vi "Sequence.Test.Load.vi"(7 "Code in":T1={"Ready"=FALSE, "DoubleOrder"=FALSE, "OrderDone"=FALSE, "AllowSingleSlot"=FALSE, "CheckDM"=FALSE, "ThresholdA"=0, "ThresholdB"=0, "Plate"=enum."Wabco", "ImgPath"=path "", "Variant"={"State"=enum."Init", "ImgPath"=path "", "WabcoPlate"="", "WabcoProduct"="", "ClientProduct"="", "ClientPlate"="", "TotalQuantity"=0, "OrderQuantity"=0, "Serial"=0, "Wabco"={"LaserJob"="", "AdditionalTxt"="037", "FactoryCode"="", "RevID"=0, "ForkID"=0, "FailuresLimit"=0, "GlobalCnt"=0, "Bank"=0, "SerialFormat"=enum."6 dig", "CoordA"={"X"=0.0, "Y"=0.0, "Angle"=0.0}, "CoordB"={"X"=0.0, "Y"=0.0, "Angle"=0.0}, "DMCconfig"=0}, "Client"={"LaserJob"="", "AdditionalTxt"="", "FactoryCode"="037", "RevID"=0, "ForkID"=0, "FailuresLimit"=0, "GlobalCnt"=0, "Bank"=0, "SerialFormat"=enum."6 dig", "CoordA"={"X"=0.0, "Y"=0.0, "Angle"=0.0}, "CoordB"={"X"=0.0, "Y"=0.0, "Angle"=0.0}, "DMCconfig"=0}}}, 8 "error in":errorcluster, 9 "#products in the machine":i32, 11 "Data in":T8) -> (0 "error out":errorcluster, 3 "Data out":T8)   [LabVIEW 2016]
uses:
  Sequence.Test.Status.ctl
  Sequence.Slot.StatusData.ctl
  Sequence.Test.Unload.Status.ctl
  Sequence.Prod.StatusData.ctl
  Sequence.Step.Status.ctl
  Sequence.Test.BreakReason.ctl
  Sequence.Code.Sets.ctl
  Sequence.PlateType.ctl
  Logger/Logger.Variant.Sets.ctl
  Station/Station.Changeover.State.vi
  Station/Station.Plate.Properties.ctl
  Sequence.Code.SerialFormat.ctl
  Drivers/V7310/LowLevel/V7310.Job.Sets.ctl
  Station/Station.ValvePosition.ctl
  Station/Station.ProductSlot.ctl
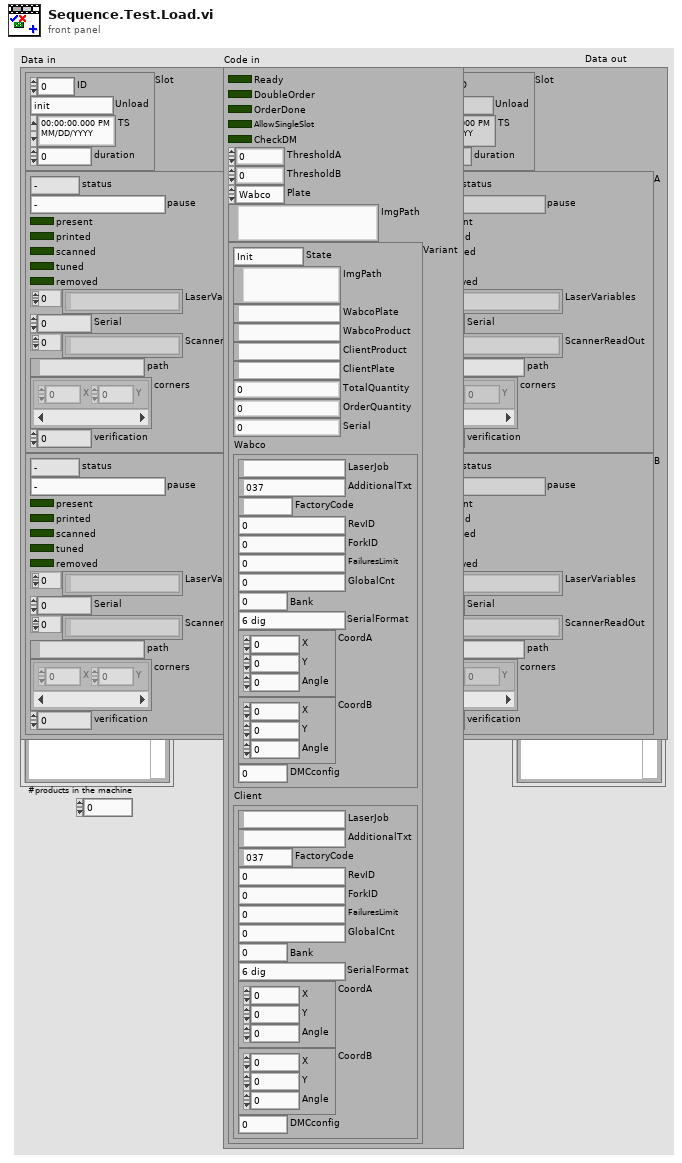
[diagram p1: front panel]
types:
  T1 = typedef "Sequence.Code.Sets.ctl" = cluster{"Ready":bool, "DoubleOrder":bool, "OrderDone":bool, "AllowSingleSlot":bool, "CheckDM":bool, "ThresholdA":u8, "ThresholdB":u8, "Plate":T2, "ImgPath":path, "Variant":T3}
  T2 = typedef "Sequence.PlateType.ctl" = enum16{"Wabco", "Client"}
  T3 = typedef "Logger.Variant.Sets.ctl" = cluster{"State":T4, "ImgPath":path, "WabcoPlate":string, "WabcoProduct":string, "ClientProduct":string, "ClientPlate":string, "TotalQuantity":u16, "OrderQuantity":u16, "Serial":i32, "Wabco":T5, "Client":T5}
  T4 = typedef "Station.Changeover.State.vi" = enum16{"Init", "Scaning", "NOK", "Wait for ack", "Ready"}
  T5 = typedef "Station.Plate.Properties.ctl" = cluster{"LaserJob":string, "AdditionalTxt":string, "FactoryCode":string, "RevID":u8, "ForkID":u8, "FailuresLimit":u16, "GlobalCnt":i32, "Bank":u8, "SerialFormat":T6, "CoordA":T7, "CoordB":T7, "DMCconfig":i32}
  T6 = typedef "Sequence.Code.SerialFormat.ctl" = enum8{"", "6 dig", "7 dig"}
  T7 = typedef "V7310.Job.Sets.ctl" = cluster{"X":dbl, "Y":dbl, "Angle":dbl}
  T8 = typedef "Sequence.Test.Status.ctl" = cluster{"Slot":T9, "A":T11, "B":T11}
  T9 = typedef "Sequence.Slot.StatusData.ctl" = cluster{"ID":i32, "Unload":T10, "TS":timestamp, "duration":u32}
  T10 = typedef "Sequence.Test.Unload.Status.ctl" = enum16{"init", "check NOK", "check OK", "wait on NOK", "wait on OK", "wait on Unload", "done"}
  T11 = typedef "Sequence.Prod.StatusData.ctl" = cluster{"status":T12, "pause":T13, "present":bool, "printed":bool, "scanned":bool, "tuned":bool, "removed":bool, "LaserVariables":string[], "Serial":i32, "ScannerReadOut":string[], "path":path, "corners":cluster{"X":i32, "Y":i32}[], "verification":u8}
  T12 = typedef "Sequence.Step.Status.ctl" = enum16{"-", "Pending", "Running", "Skipped", "Passed", "Failed", "Done", "Error", "Aborted", "Stopped"}
  T13 = typedef "Sequence.Test.BreakReason.ctl" = enum16{"-", "NOK container", "OK container", "Rev empty", "Rev missing", "Rev wrong", "Fork missing", "Fork wrong", "NOK limit", "Unload failure", "Single slot", "Part done", "Err: Prod move work", "Err: Prod move home", "Err: Prod lift work", "Err: Prod lift home", "Err: Prod Arm Work", "Err: Prod Arm NOK", "Err: Prod Arm OK", "Err: Prod NOK suck", "Err: Prod NOK drop", "Err: Prod OK missing", "Err: Prod OK suck", "Err: Prod OK drop"}
  T14 = typedef "Station.ValvePosition.ctl" = enum16{"Home", "Work"}
  T15 = typedef "FestoCPX.Station.RevolverID.ctl" = cluster{"ID":u8, "1":bool, "2":bool, "3":bool, "4":bool, "5":bool}
  T16 = typedef "Station.ProductSlot.ctl" = enum8{"A", "B"}
  T17 = typedef "Sequence.SerialsFglb.StatusFlags.ctl" = cluster{"Global":bool, "NokLimit":bool, "PartDone":bool, "Completed":bool}
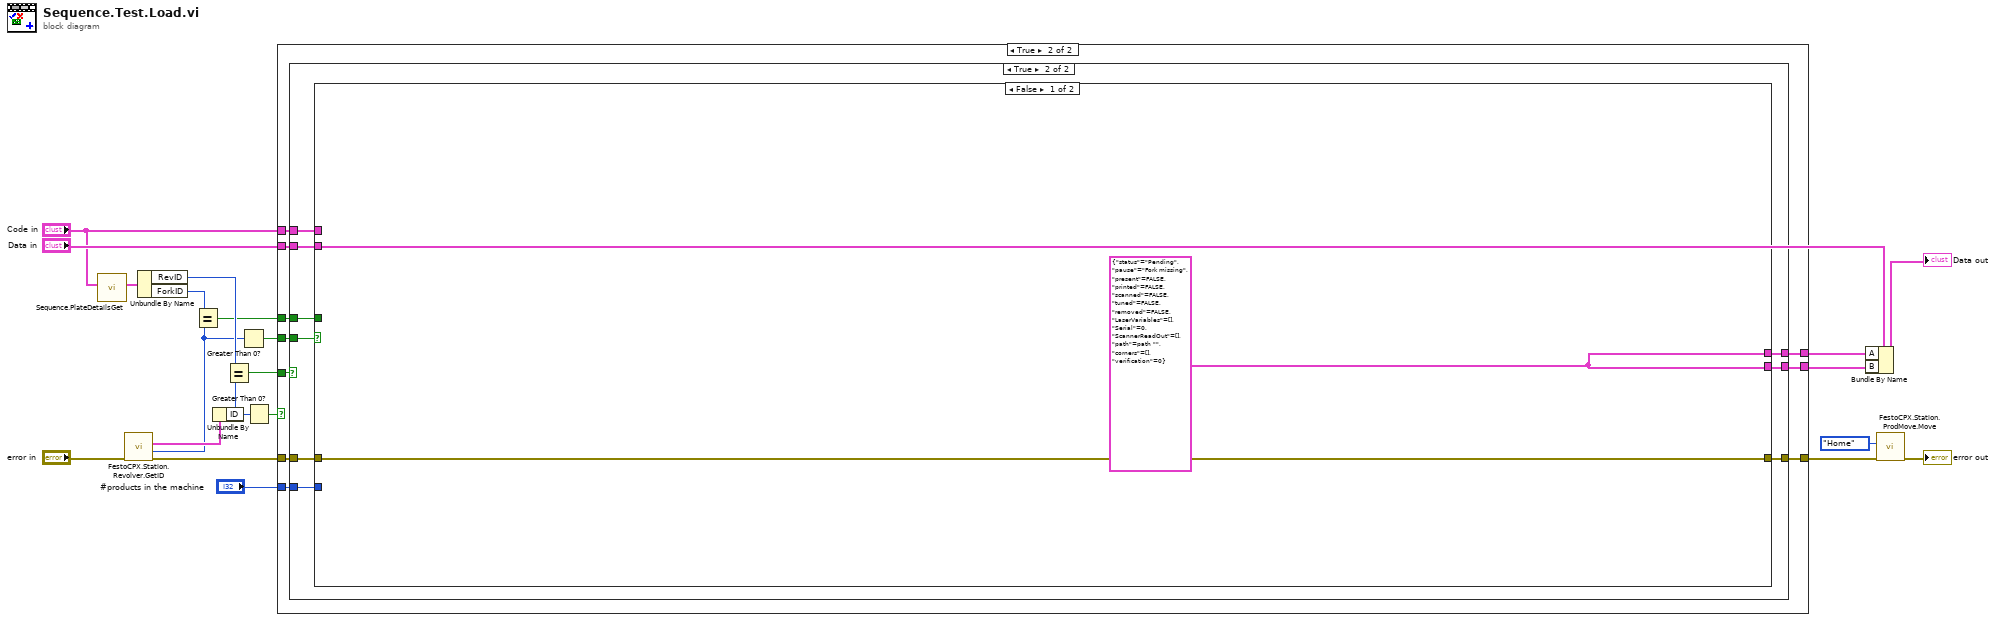
[diagram p0: block diagram]
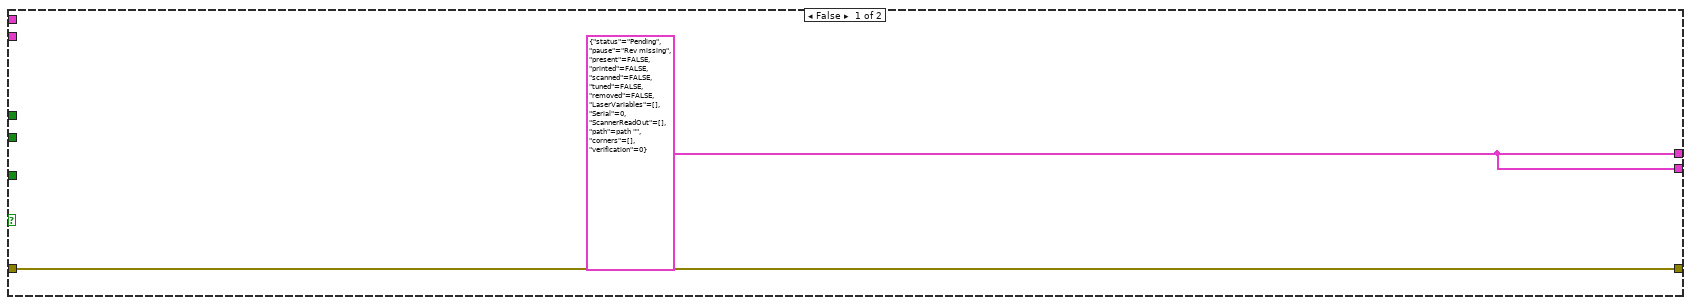
[diagram p2: hidden frame]
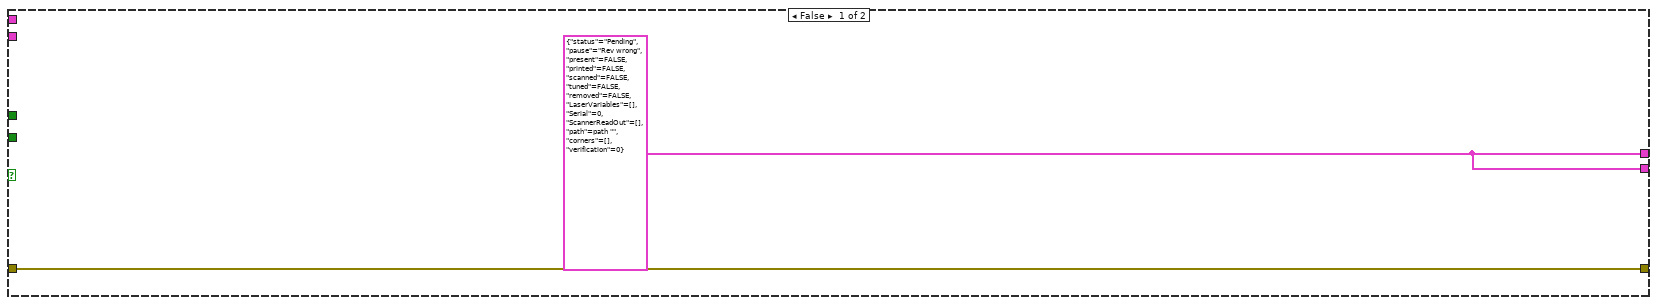
[diagram p3: hidden frame]
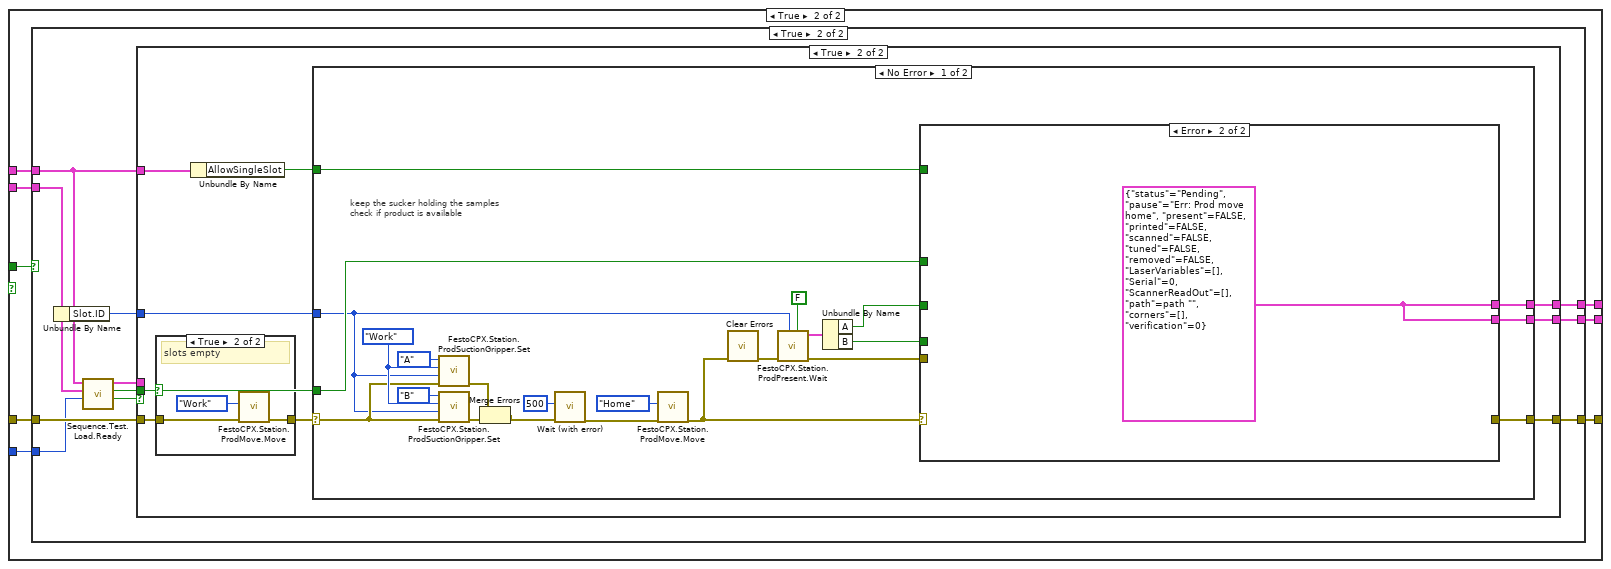
[diagram p4: hidden frame]
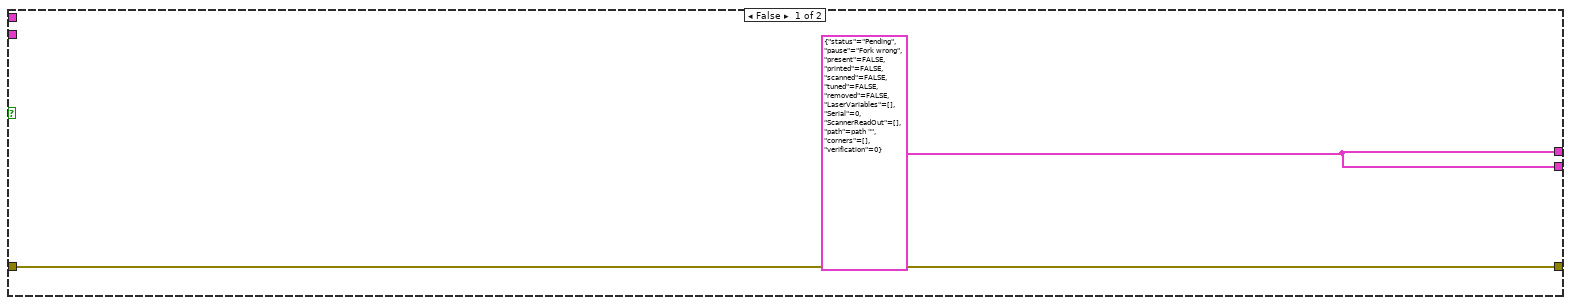
[diagram p5: hidden frame]
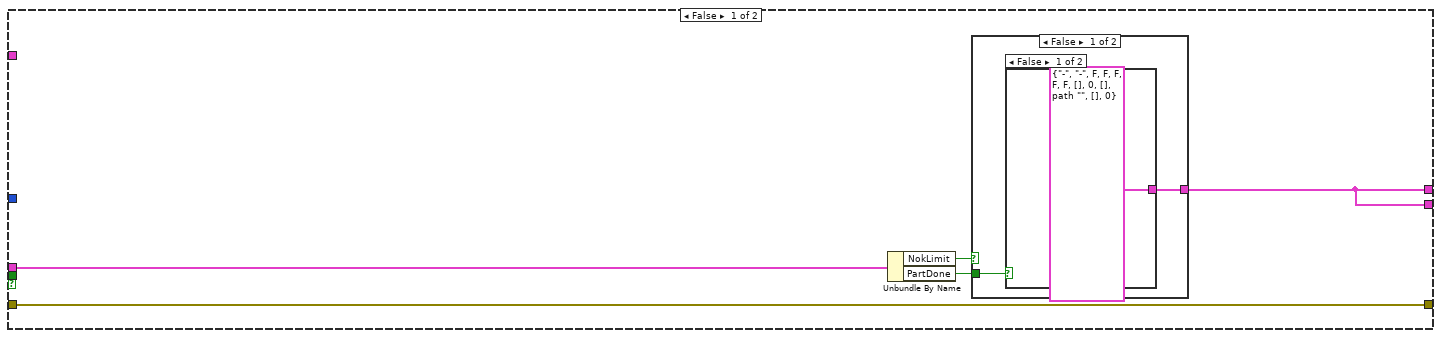
[diagram p6: hidden frame]
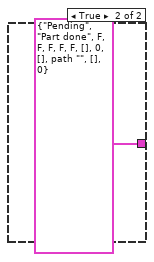
[diagram p7: hidden frame]
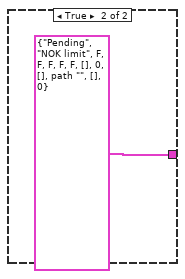
[diagram p8: hidden frame]
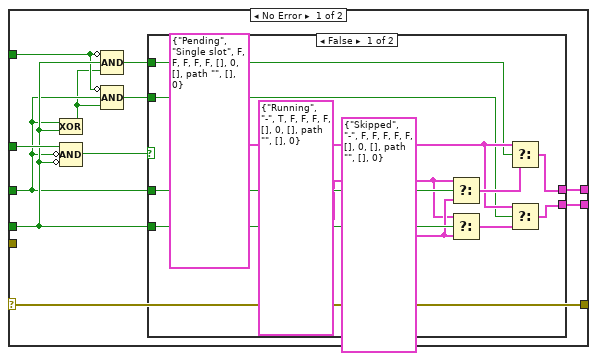
[diagram p9: hidden frame]
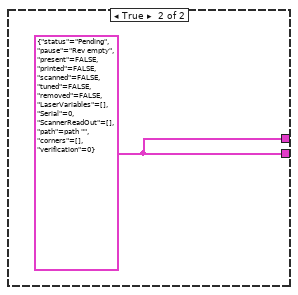
[diagram p10: hidden frame]
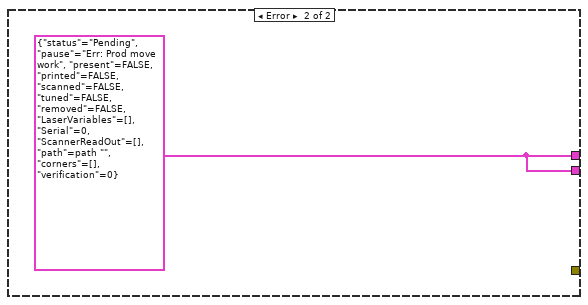
[diagram p11: hidden frame]
diagram:
  n1 = call "Sequence.PlateDetailsGet.vi"("Code in"="Code in") -> ("PlateDetails"=w3:T5)  [unwired: 9 in, 1 out]
  n2 = call "FestoCPX.Station.Revolver.GetID.vi"("error in"="error in") -> ("error out"=w16:errorcluster, "ForkID"=w8:u8, "RevID"=w15:T15)  [unwired: 8 in]
  n3 = Unbundle By Name(w3) -> ("RevID"=w10:u8, "ForkID"=w11:u8)
  n4 = Equal?(x=w11, y=w8) -> (x = y?=w9:bool)
  n5 = Unbundle By Name(w15) -> ("ID"=w13:u8)
  n6 = Equal?(x=w10, y=w13) -> (x = y?=w12:bool)
  n7 = Greater Than 0?(x=w8) -> (x > 0?=w7:bool)
  n8 = Greater Than 0?(x=w13) -> (x > 0?=w14:bool)
  n9 = case shown="True" w14 {
    tunnel: [w23 w33] -> w20
    tunnel: [w23 w32] -> w19
    tunnel: [w22 w31] -> w5
    tunnel: "Data in" -> [_ w30]
    tunnel: "Code in" -> [_ w29]
    tunnel: w16 -> [w22 w28]
    tunnel: w12 -> [_ w27]
    tunnel: w9 -> [_ w26]
    tunnel: w7 -> [_ w25]
    tunnel: "#products in the machine" -> [_ w24]
    frame False {
      w23 = T11 {"status"=enum."Pending", "pause"=enum."Rev missing", "present"=FALSE, "printed"=FALSE, "scanned"=FALSE, "tuned"=FALSE, "removed"=FALSE, "LaserVariables"=[], "Serial"=0, "ScannerReadOut"=[], "path"=path "", "corners"=[], "verification"=0} ("A")
    }
    frame True {
      n10 = case shown="True" w27 {
        tunnel: [w35 w44] -> w33
        tunnel: [w35 w43] -> w32
        tunnel: [w34 w42] -> w31
        tunnel: w30 -> [_ w41]
        tunnel: w29 -> [_ w39]
        tunnel: w28 -> [w34 w40]
        tunnel: w26 -> [_ w38]
        tunnel: w25 -> [_ w37]
        tunnel: w24 -> [_ w36]
        frame False {
          w35 = T11 {"status"=enum."Pending", "pause"=enum."Rev wrong", "present"=FALSE, "printed"=FALSE, "scanned"=FALSE, "tuned"=FALSE, "removed"=FALSE, "LaserVariables"=[], "Serial"=0, "ScannerReadOut"=[], "path"=path "", "corners"=[], "verification"=0} ("A")
        }
        frame True {
          n11 = case shown="False" w37 {
            tunnel: [w46 w54] -> w44
            tunnel: [w46 w53] -> w43
            tunnel: [w45 w52] -> w42
            tunnel: w41 -> [_ w51]
            tunnel: w40 -> [w45 w50]
            tunnel: w39 -> [_ w49]
            tunnel: w38 -> [_ w48]
            tunnel: w36 -> [_ w47]
            frame False {
              w46 = T11 {"status"=enum."Pending", "pause"=enum."Fork missing", "present"=FALSE, "printed"=FALSE, "scanned"=FALSE, "tuned"=FALSE, "removed"=FALSE, "LaserVariables"=[], "Serial"=0, "ScannerReadOut"=[], "path"=path "", "corners"=[], "verification"=0} ("A")
            }
            frame True {
              n12 = case shown="True" w48 {
                tunnel: [w56 w67] -> w54
                tunnel: [w56 w66] -> w53
                tunnel: [w55 w65] -> w52
                tunnel: w51 -> [_ w63]
                tunnel: w50 -> [w55 w62]
                tunnel: w49 -> [_ w59]
                tunnel: w47 -> [_ w57]
                frame False {
                  w56 = T11 {"status"=enum."Pending", "pause"=enum."Fork wrong", "present"=FALSE, "printed"=FALSE, "scanned"=FALSE, "tuned"=FALSE, "removed"=FALSE, "LaserVariables"=[], "Serial"=0, "ScannerReadOut"=[], "path"=path "", "corners"=[], "verification"=0} ("A")
                }
                frame True {
                  n13 = Unbundle By Name(w63) -> ("Slot.ID"=w64:i32)
                  n14 = call "Sequence.Test.Load.Ready.vi"("#products in the machine"=w57, "Data in"=w63, "Code in"=w59) -> ("Ready"=w61:bool, "Loaded"=w60:bool, "StatusFlags"=w58:T17)  [unwired: 6 in]
                  n15 = case shown="True" w61 {
                    tunnel: [w72 w86] -> w67
                    tunnel: [w72 w85] -> w66
                    tunnel: [w69 w78] -> w65
                    tunnel: w64 -> [_ w82]
                    tunnel: w62 -> [w69 w84]
                    tunnel: w60 -> [_ w83]
                    tunnel: w59 -> [_ w81]
                    tunnel: w58 -> [w68 _]
                    frame False {
                      n16 = Unbundle By Name(w68) -> ("NokLimit"=w71:bool, "PartDone"=w70:bool)
                      n17 = case shown="False" w71 {
                        tunnel: [w74 T11 {"status"=enum."Pending", "pause"=enum."NOK limit", "present"=FALSE, "printed"=FALSE, "scanned"=FALSE, "tuned"=FALSE, "removed"=FALSE, "LaserVariables"=[], "Serial"=0, "ScannerReadOut"=[], "path"=path "", "corners"=[], "verification"=0} ("A")] -> w72
                        tunnel: w70 -> [w73 _]
                        frame False {
                          n18 = case shown="False" w73 {
                            tunnel: [T11 {"status"=enum."-", "pause"=enum."-", "present"=FALSE, "printed"=FALSE, "scanned"=FALSE, "tuned"=FALSE, "removed"=FALSE, "LaserVariables"=[], "Serial"=0, "ScannerReadOut"=[], "path"=path "", "corners"=[], "verification"=0} ("A") T11 {"status"=enum."Pending", "pause"=enum."Part done", "present"=FALSE, "printed"=FALSE, "scanned"=FALSE, "tuned"=FALSE, "removed"=FALSE, "LaserVariables"=[], "Serial"=0, "ScannerReadOut"=[], "path"=path "", "corners"=[], "verification"=0} ("A")] -> w74
                            frame False {
                            }
                            frame True {
                            }
                          }
                        }
                        frame True {
                        }
                      }
                    }
                    frame True {
                      n19 = case shown="True" w83 {
                        tunnel: w84 -> [w135 w137]
                        tunnel: [w135 w136] -> w79
                        frame False {
                          # "product already loaded"
                        }
                        frame True {
                          # "slots empty"
                          n20 = call "FestoCPX.Station.ProdMove.Move.vi"("error in"=w137, "Position"=Station.ValvePosition."Work") -> ("error out"=w136:errorcluster)  [unwired: 8 in, 1 out]
                        }
                      }
                      n21 = Unbundle By Name(w81) -> ("AllowSingleSlot"=w80:bool)
                      n22 = case shown="No Error" w79 {
                        selector: w79 -> [w94 _]
                        tunnel: [w109 w134] -> w86
                        tunnel: [w108 w134] -> w85
                        tunnel: w83 -> [w104 _]
                        tunnel: w82 -> [w90 _]
                        tunnel: w80 -> [w93 _]
                        tunnel: [w95 _] -> w78
                        frame No Error {
                          w105 = Station.ValvePosition."Work" ("Position")
                          # "keep the sucker holding the samples\ncheck if product is available"
                          n23 = call "FestoCPX.Station.ProdSuctionGripper.Set.vi"("error in"=w94, "Sucker (0: Final)"=w90, "Position"=w105, "Slot"=Station.ProductSlot."A") -> ("error out"=w103:errorcluster)  [unwired: 6 in, 1 out]
                          n24 = call "FestoCPX.Station.ProdSuctionGripper.Set.vi"("error in"=w94, "Sucker (0: Final)"=w90, "Position"=w105, "Slot"=Station.ProductSlot."B") -> ("error out"=w102:errorcluster)  [unwired: 6 in, 1 out]
                          n25 = Merge Errors(w103, w102) -> (w89:errorcluster)
                          n26 = call "Wait (with error).vi"("error in (no error)"=w89, "milliseconds to wait"=u32 500) -> ("error out"=w97:errorcluster)  [unwired: 8 in, 1 out]
                          n27 = call "FestoCPX.Station.ProdMove.Move.vi"("error in"=w97, "Position"=Station.ValvePosition."Home") -> ("error out"=w87:errorcluster)  [unwired: 8 in, 1 out]
                          n28 = call <vilib>:"Clear Errors.vi"("error in (no error)"=w87) -> ("error out"=w96:errorcluster)  [unwired: 5 in, 1 out]
                          n29 = call "FestoCPX.Station.ProdPresent.Wait.vi"("AllowSingleSlot"=FALSE, "SuckerID (0: Final)"=w90, "error in"=w96) -> ("error out"=w91:errorcluster, "Present.SuckerID"=w100:cluster{"A":bool, "B":bool})  [unwired: 7 in]
                          n30 = Unbundle By Name(w100) -> ("A"=w92:bool, "B"=w99:bool)
                          n31 = case shown="Error" w87 {
                            selector: w87 -> [w110 _]
                            tunnel: [w120 w133] -> w109
                            tunnel: [w119 w133] -> w108
                            tunnel: w92 -> [w112 _]
                            tunnel: w99 -> [w116 _]
                            tunnel: w104 -> [w118 _]
                            tunnel: w93 -> [w113 _]
                            tunnel: [w110 _] -> w95
                            tunnel: w91 -> [_ _]
                            frame No Error {
                              n32 = Compound Arithmetic op=XOR(w112, w116) -> (w111:bool)
                              n33 = Compound Arithmetic op=AND(w118, invert w112, invert w116) -> (w117:bool)
                              n34 = Compound Arithmetic op=AND(invert w113, w116, w111) -> (w115:bool)
                              n35 = Compound Arithmetic op=AND(invert w113, w112, w111) -> (w114:bool)
                              n36 = case shown="False" w117 {
                                tunnel: [w127 w132] -> w120
                                tunnel: [w125 w132] -> w119
                                tunnel: w112 -> [w131 _]
                                tunnel: w116 -> [w130 _]
                                tunnel: w115 -> [w122 _]
                                tunnel: w114 -> [w121 _]
                                frame False {
                                w123 = T11 {"status"=enum."Pending", "pause"=enum."Single slot", "present"=FALSE, "printed"=FALSE, "scanned"=FALSE, "tuned"=FALSE, "removed"=FALSE, "LaserVariables"=[], "Serial"=0, "ScannerReadOut"=[], "path"=path "", "corners"=[], "verification"=0} ("A")
                                w129 = T11 {"status"=enum."Skipped", "pause"=enum."-", "present"=FALSE, "printed"=FALSE, "scanned"=FALSE, "tuned"=FALSE, "removed"=FALSE, "LaserVariables"=[], "Serial"=0, "ScannerReadOut"=[], "path"=path "", "corners"=[], "verification"=0} ("A")
                                w128 = T11 {"status"=enum."Running", "pause"=enum."-", "present"=TRUE, "printed"=FALSE, "scanned"=FALSE, "tuned"=FALSE, "removed"=FALSE, "LaserVariables"=[], "Serial"=0, "ScannerReadOut"=[], "path"=path "", "corners"=[], "verification"=0} ("A")
                                n37 = Select(t=w128, s=w131, f=w129) -> (s? t:f=w124:T11)
                                n38 = Select(t=w128, s=w130, f=w129) -> (s? t:f=w126:T11)
                                n39 = Select(t=w123, s=w122, f=w124) -> (s? t:f=w127:T11)
                                n40 = Select(t=w123, s=w121, f=w126) -> (s? t:f=w125:T11)
                                }
                                frame True {
                                w132 = T11 {"status"=enum."Pending", "pause"=enum."Rev empty", "present"=FALSE, "printed"=FALSE, "scanned"=FALSE, "tuned"=FALSE, "removed"=FALSE, "LaserVariables"=[], "Serial"=0, "ScannerReadOut"=[], "path"=path "", "corners"=[], "verification"=0} ("A")
                                }
                              }
                            }
                            frame Error {
                              w133 = T11 {"status"=enum."Pending", "pause"=enum."Err: Prod move home", "present"=FALSE, "printed"=FALSE, "scanned"=FALSE, "tuned"=FALSE, "removed"=FALSE, "LaserVariables"=[], "Serial"=0, "ScannerReadOut"=[], "path"=path "", "corners"=[], "verification"=0} ("A")
                            }
                          }
                        }
                        frame Error {
                          w134 = T11 {"status"=enum."Pending", "pause"=enum."Err: Prod move work", "present"=FALSE, "printed"=FALSE, "scanned"=FALSE, "tuned"=FALSE, "removed"=FALSE, "LaserVariables"=[], "Serial"=0, "ScannerReadOut"=[], "path"=path "", "corners"=[], "verification"=0} ("A")
                        }
                      }
                    }
                  }
                }
              }
            }
          }
        }
      }
    }
  }
  n41 = Bundle By Name(cluster="Data in", "A"=w20, "B"=w19) -> (→"Data out":T8)
  n42 = call "FestoCPX.Station.ProdMove.Move.vi"("error in"=w5, "Position"=Station.ValvePosition."Home") -> ("error out"=→"error out":errorcluster)  [unwired: 8 in, 1 out]
